vi "Reset Timer Method.vi"(8 "error in (no error)":errorcluster) -> (0 "error out":errorcluster, 1 "New Elapsed Time (s)":dbl, 2 "New Time Stamp":dbl)   [LabVIEW 2013]
doc: "This sub-VI implements the Rezero function of the car wash timer. The Elapsed Time and Last Time Stamp values are state variables and are stored externally to this sub-VI. The New Time Stamp and New Elapsed Time will overwrite the stored values."
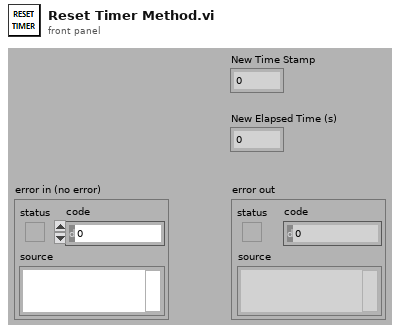
[diagram p1: front panel]
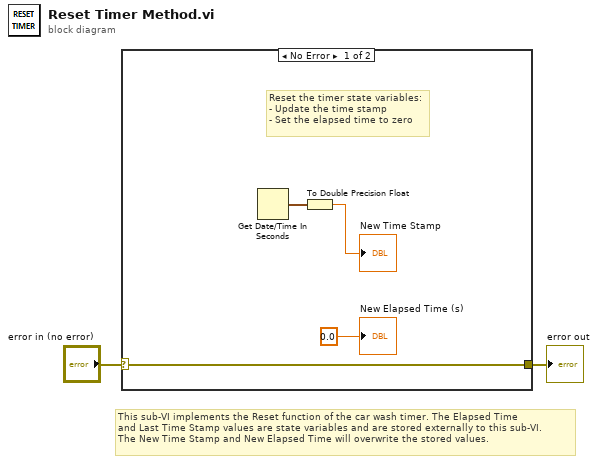
[diagram p0: block diagram]
diagram:
  # "This sub-VI implements the Reset function of the car wash timer. The Elapsed Time \nand Last Time Stamp values are state variables and are stored externally to this sub-VI.  \nThe New Time Stamp and New Elapsed Time will overwrite the stored values."
  n1 = case shown="No Error" "error in (no error)" {
    selector: "error in (no error)" -> [w3 w7]
    tunnel: [w3 w7] -> w1
    frame No Error {
      # "Reset the timer state variables:\n- Update the time stamp\n- Set the elapsed time to zero"
      n2 = Get Date/Time In Seconds() -> (seconds since 1Jan1904=w6:timestamp)
      n3 = To Double Precision Float(number=w6) -> (double precision float=→"New Time Stamp":dbl)
      "New Elapsed Time (s)" <- 0.0 ("Reset Elapsed Time (s)")
    }
    frame Error {
    }
  }
  "error out" <- w1
